vi "templates get user info from username.vi"(8 "error in (no error)":errorcluster, 10 "Username (\"\")":string, 11 "Connection Refnum":T1) -> (0 "error out":errorcluster, 1 "Email":string, 2 "First Last":string, 3 "Connection Refnum":T1)   [LabVIEW 2011]
uses:
  Summitek EXT/ODBC/SQL Controls/Connection Refnum.ctl
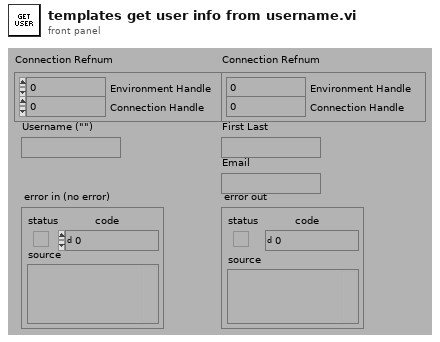
[diagram p1: front panel]
types:
  T1 = typedef "Connection Refnum.ctl" = cluster{"Environment Handle":i32, "Connection Handle":i32}
  T2 = typedef "User Record.ctl" = cluster{"ixUser":i32, "sxUsername":string, "sLastName":string, "sFirstName":string, "sEmail":string, "sPassword":string, "tLoginTime":timestamp, "sLoginComputer":string, "fAdministrator":bool, "fRunSequences":bool, "fModifySequences":bool, "fRunScenarios":bool, "fModifyScenarios":bool, "fModifyTemplates":bool, "fModifyUsers":bool, "fModifyStations":bool, "fModifyFields":bool}
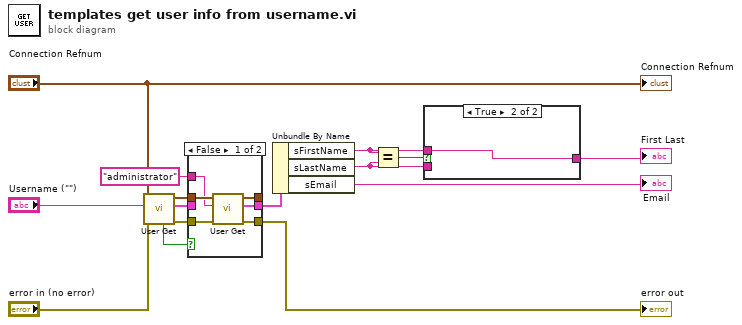
[diagram p0: block diagram]
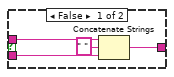
[diagram p2: hidden frame]
diagram:
  n1 = call "User Get.vi"("error in (no error)"="error in (no error)", "sxUsername (\"\")"="Username (\"\")", "Connection Refnum"="Connection Refnum") -> ("error out"=w15:errorcluster, "User"=w13:T2, "Connection Refnum"=w11:T1, "Data Present?"=w14:bool)  [unwired: 5 out]
  n2 = case shown="False" w14 {
    tunnel: w15 -> [w20 w24]
    tunnel: [w19 w24] -> w5
    tunnel: [w16 w23] -> w12
    tunnel: w13 -> [_ w23]
    tunnel: [w18 w22] -> _
    tunnel: w11 -> [w21 w22]
    tunnel: "administrator" -> [w17 _]
    frame False {
      n3 = call "User Get.vi"("error in (no error)"=w20, "sxUsername (\"\")"=w17, "Connection Refnum"=w21) -> ("error out"=w19:errorcluster, "User"=w16:T2, "Connection Refnum"=w18:T1)  [unwired: 6 out]
    }
    frame True {
    }
  }
  "error out" <- w5
  n4 = Unbundle By Name(w12) -> ("sFirstName"=w3:string, "sLastName"=w2:string, "sEmail"=→"Email":string)
  n5 = Equal?(x=w3, y=w2) -> (x = y?=w1:bool)
  n6 = case shown="True" w1 {
    tunnel: [w27 w29] -> w9
    tunnel: w3 -> [w26 w29]
    tunnel: w2 -> [w25 _]
    frame False {
      n7 = Concatenate Strings(w26, " ", w25) -> (w27:string)
    }
    frame True {
    }
  }
  "First Last" <- w9
  "Connection Refnum" <- "Connection Refnum"
